vi "Demo_PlotMusic.vi"() -> ()   [LabVIEW 2021, in "RocketPlotDemo.lvlib"]
uses:
  Demo/RocketPlotDemo.lvlib
  TypeDefs/plot load data V2.ctl
  TypeDefs/plot properties V2.ctl
  TypeDefs/plot attributes V2.ctl
  TypeDefs/Plot scale axis properties.ctl
  TypeDefs/Plot general properties.ctl
  Classes/RocketPlotHandle/SubVIs/Init Options.ctl
  TypeDefs/TimeZone.ctl
  Classes/BjusticePlotHandle/Type.ctl
  <vilib>/sound2/lvsound2.llb/Sampling Mode.ctl
  Classes/RocketPlotPanel/RocketPlotPanel.lvclass/RocketPlotPanel.ctl
  4dfea61d-788a-4186-b191-4cde70d6fed2.vi
  966c8643-725a-46bd-9dd0-b91467cf4ddd.vi
  eb0507fd-03f2-4275-8513-22fa9a77d05c.vi
  2cc444ce-eb93-4e53-95b9-bbf802b1ec09.vi
  0323ff41-b8ad-4ed8-8c31-07cadd3001fa.vi
  44d01159-0067-4c41-b020-b8d23d8c44ab.vi
  286f873d-ace6-4cc1-b7d0-d8c3bbebe2d8.vi
  d8c1f50c-a031-4c7b-bbc9-5a9a3e4568ff.vi
  d49b8d8d-7917-4e09-824a-362aaf82a6cf.vi
  35cc1419-e3af-44ec-a6f0-6af3754db062.vi
  Classes/RocketPlotPanel/Read RocketPlotHandle.vi
  <userlib>/bjustice/Ring Buffer for Time Series Data Strict Accessor/Unix time epoch/Unix_Epoch_in_Labview.vi
  0323ff41-b8ad-4ed8-8c31-07cadd3001fa.vi/4c2a6c61-f100-483c-8a49-51e57025a24c.vi
  0323ff41-b8ad-4ed8-8c31-07cadd3001fa.vi/e57bc314-87c7-4952-9bc8-929005dac297.vi
  44d01159-0067-4c41-b020-b8d23d8c44ab.vi/4c2a6c61-f100-483c-8a49-51e57025a24c.vi
  44d01159-0067-4c41-b020-b8d23d8c44ab.vi/e57bc314-87c7-4952-9bc8-929005dac297.vi
  <userlib>/bjustice/Ring Buffer for Time Series Data/API Poly.vi
  <userlib>/bjustice/Ring Buffer for Time Series Data/API/Write Array.vi
  d8c1f50c-a031-4c7b-bbc9-5a9a3e4568ff.vi/f2df9050-0eef-46c6-aff6-3ce3a8893ea5.vi
  35cc1419-e3af-44ec-a6f0-6af3754db062.vi/f2df9050-0eef-46c6-aff6-3ce3a8893ea5.vi
  <userlib>/bjustice/Ring Buffer for Time Series Data/SubVIs/Split Values Array.vi
  <userlib>/bjustice/Ring Buffer for Time Series Data/SubVIs/Replace Values Array Multiple Timestamps.vi
  d8c1f50c-a031-4c7b-bbc9-5a9a3e4568ff.vi/f2df9050-0eef-46c6-aff6-3ce3a8893ea5.vi/63c583a5-c20f-4aba-9c90-661423dee4c4.vi
  d8c1f50c-a031-4c7b-bbc9-5a9a3e4568ff.vi/f2df9050-0eef-46c6-aff6-3ce3a8893ea5.vi/52385341-3d9c-45d2-aff5-e082a4793eb1.vi
  d8c1f50c-a031-4c7b-bbc9-5a9a3e4568ff.vi/f2df9050-0eef-46c6-aff6-3ce3a8893ea5.vi/37f29efa-f142-46b1-a185-f0098a95fbb6.vi
  d8c1f50c-a031-4c7b-bbc9-5a9a3e4568ff.vi/f2df9050-0eef-46c6-aff6-3ce3a8893ea5.vi/84b3d231-9afe-4b6e-afae-e0be43a31e4e.vi
  d8c1f50c-a031-4c7b-bbc9-5a9a3e4568ff.vi/f2df9050-0eef-46c6-aff6-3ce3a8893ea5.vi/c726271c-fc36-4bb7-8553-8945ec40c1cd.vi
  d8c1f50c-a031-4c7b-bbc9-5a9a3e4568ff.vi/f2df9050-0eef-46c6-aff6-3ce3a8893ea5.vi/a7b1d944-dc88-46f5-9d3e-305d46bbe1f6.vi
  d8c1f50c-a031-4c7b-bbc9-5a9a3e4568ff.vi/f2df9050-0eef-46c6-aff6-3ce3a8893ea5.vi/8abc4a6e-a1d2-4e85-879b-517e0ab55733.vi
  d8c1f50c-a031-4c7b-bbc9-5a9a3e4568ff.vi/f2df9050-0eef-46c6-aff6-3ce3a8893ea5.vi/bd347357-b475-4a03-9ac5-3b85ef11aecc.vi
  d8c1f50c-a031-4c7b-bbc9-5a9a3e4568ff.vi/f2df9050-0eef-46c6-aff6-3ce3a8893ea5.vi/391b36e9-a702-45e4-9499-3914f8833a58.vi
  d8c1f50c-a031-4c7b-bbc9-5a9a3e4568ff.vi/f2df9050-0eef-46c6-aff6-3ce3a8893ea5.vi/44155b33-c915-49ce-9e44-a66693aa70dd.vi
  d8c1f50c-a031-4c7b-bbc9-5a9a3e4568ff.vi/f2df9050-0eef-46c6-aff6-3ce3a8893ea5.vi/36977d53-dbe0-4dbc-b2ac-3dea4345b868.vi
  35cc1419-e3af-44ec-a6f0-6af3754db062.vi/f2df9050-0eef-46c6-aff6-3ce3a8893ea5.vi/63c583a5-c20f-4aba-9c90-661423dee4c4.vi
  35cc1419-e3af-44ec-a6f0-6af3754db062.vi/f2df9050-0eef-46c6-aff6-3ce3a8893ea5.vi/52385341-3d9c-45d2-aff5-e082a4793eb1.vi
  35cc1419-e3af-44ec-a6f0-6af3754db062.vi/f2df9050-0eef-46c6-aff6-3ce3a8893ea5.vi/37f29efa-f142-46b1-a185-f0098a95fbb6.vi
  35cc1419-e3af-44ec-a6f0-6af3754db062.vi/f2df9050-0eef-46c6-aff6-3ce3a8893ea5.vi/84b3d231-9afe-4b6e-afae-e0be43a31e4e.vi
  35cc1419-e3af-44ec-a6f0-6af3754db062.vi/f2df9050-0eef-46c6-aff6-3ce3a8893ea5.vi/c726271c-fc36-4bb7-8553-8945ec40c1cd.vi
  35cc1419-e3af-44ec-a6f0-6af3754db062.vi/f2df9050-0eef-46c6-aff6-3ce3a8893ea5.vi/a7b1d944-dc88-46f5-9d3e-305d46bbe1f6.vi
  35cc1419-e3af-44ec-a6f0-6af3754db062.vi/f2df9050-0eef-46c6-aff6-3ce3a8893ea5.vi/8abc4a6e-a1d2-4e85-879b-517e0ab55733.vi
  35cc1419-e3af-44ec-a6f0-6af3754db062.vi/f2df9050-0eef-46c6-aff6-3ce3a8893ea5.vi/bd347357-b475-4a03-9ac5-3b85ef11aecc.vi
  35cc1419-e3af-44ec-a6f0-6af3754db062.vi/f2df9050-0eef-46c6-aff6-3ce3a8893ea5.vi/391b36e9-a702-45e4-9499-3914f8833a58.vi
  35cc1419-e3af-44ec-a6f0-6af3754db062.vi/f2df9050-0eef-46c6-aff6-3ce3a8893ea5.vi/44155b33-c915-49ce-9e44-a66693aa70dd.vi
  35cc1419-e3af-44ec-a6f0-6af3754db062.vi/f2df9050-0eef-46c6-aff6-3ce3a8893ea5.vi/36977d53-dbe0-4dbc-b2ac-3dea4345b868.vi
  <userlib>/bjustice/Ring Buffer for Time Series Data/SubVIs/Enforce array size multiple timestamps.vi
  Classes/BjusticePlotHandle/BjusticePlotHandle.lvclass
  C:/Users/bjustice/Documents/GitHub/BluePlot/Source/Classes/RocketPlotHandle/RocketPlotHandle.lvclass
  Classes/RocketPlotPanel/RocketPlotPanel.lvclass
  C:/Program Files/National Instruments/LabVIEW 2021/vi.lib/IlluminatedG/IG OOPanel/OOPanel/Panel/Panel.lvclass
  <vilib>/sound2/lvsound2.llb/Sound File Info (path).vi
  <vilib>/sound2/lvsound2.llb/Sound File Read Open.vi
  <vilib>/sound2/lvsound2.llb/Sound Output Set Volume (Single).vi
  Classes/RocketPlotHandle/Load PlotConfig.vi
  Classes/RocketPlotHandle/Get PlotConfig.vi
  <vilib>/sound2/lvsound2.llb/Sound File Read (DBL).vi
  <vilib>/Utility/error.llb/Error Cluster From Error Code.vi
  <vilib>/sound2/lvsound2.llb/Sound Output Write (DBL).vi
  Classes/RocketPlotHandle/RocketPlotHandle.lvclass
  RocketPlot.lvlib
  <userlib>/bjustice/Ring Buffer for Time Series Data Strict Accessor/Ring Buffer Strict Accessor.lvlib
  <vilib>/IlluminatedG/IG OOPanel/OOPanel/Manager/Manager.lvclass
panel:
  in  "volume":dbl=100.0
  out "total number of samples/ch":u32
  out "Current Iteration":i32
  out "Current Data":waveform(dbl)[](graph)
  in  "load config":bool
  in  "get config":bool
  out "time to plot":dbl
  out "Subscribed names":i32(listbox)
  in  "Plot config":T1={"plots"=[], "X-axis"={"Name Label.Text"="", "Style"=0, "Tick Colors:Minor Tick Color"=0, "Tick Colors:Tick Color"=0, "Marker Colors:Text Color"=0, "Grid Colors:Major Color"=0, "Grid Colors:Minor Color"=0, "Mapping Mode"=0, "Flipped"=FALSE, "Name Label.Visible"=FALSE, "Name Label.Text Colors:Text Color"=0, "Scale Fit"=0, "Range:Maximum"=0.0, "Range:Minimum"=0.0, "Offset and Multiplier:Multiplier"=0.0, "Offset and Multiplier:Offset"=0.0, "Name Label.Font:Size"=0, "Marker.Font:Size"=0, "Uniform Marker Spacing?"=TRUE, "Format String"=""}, "Y-axes"=[], "General"={"Title"="", "Time to Plot"=1800.0, "Title.Visible"=FALSE, "Sidebar.Visible"=FALSE, "Plot Area:Colors:BG Color"=0, "X Scale.Plot Name"="", "X Scale.Use Plot Name"=FALSE}} {"General"."Time to Plot" format="%<%M:%S>t"}
  # "Documentation and user guide:"
  # "https://github.com/justiceb/BluePlot/blob/main/README.md"
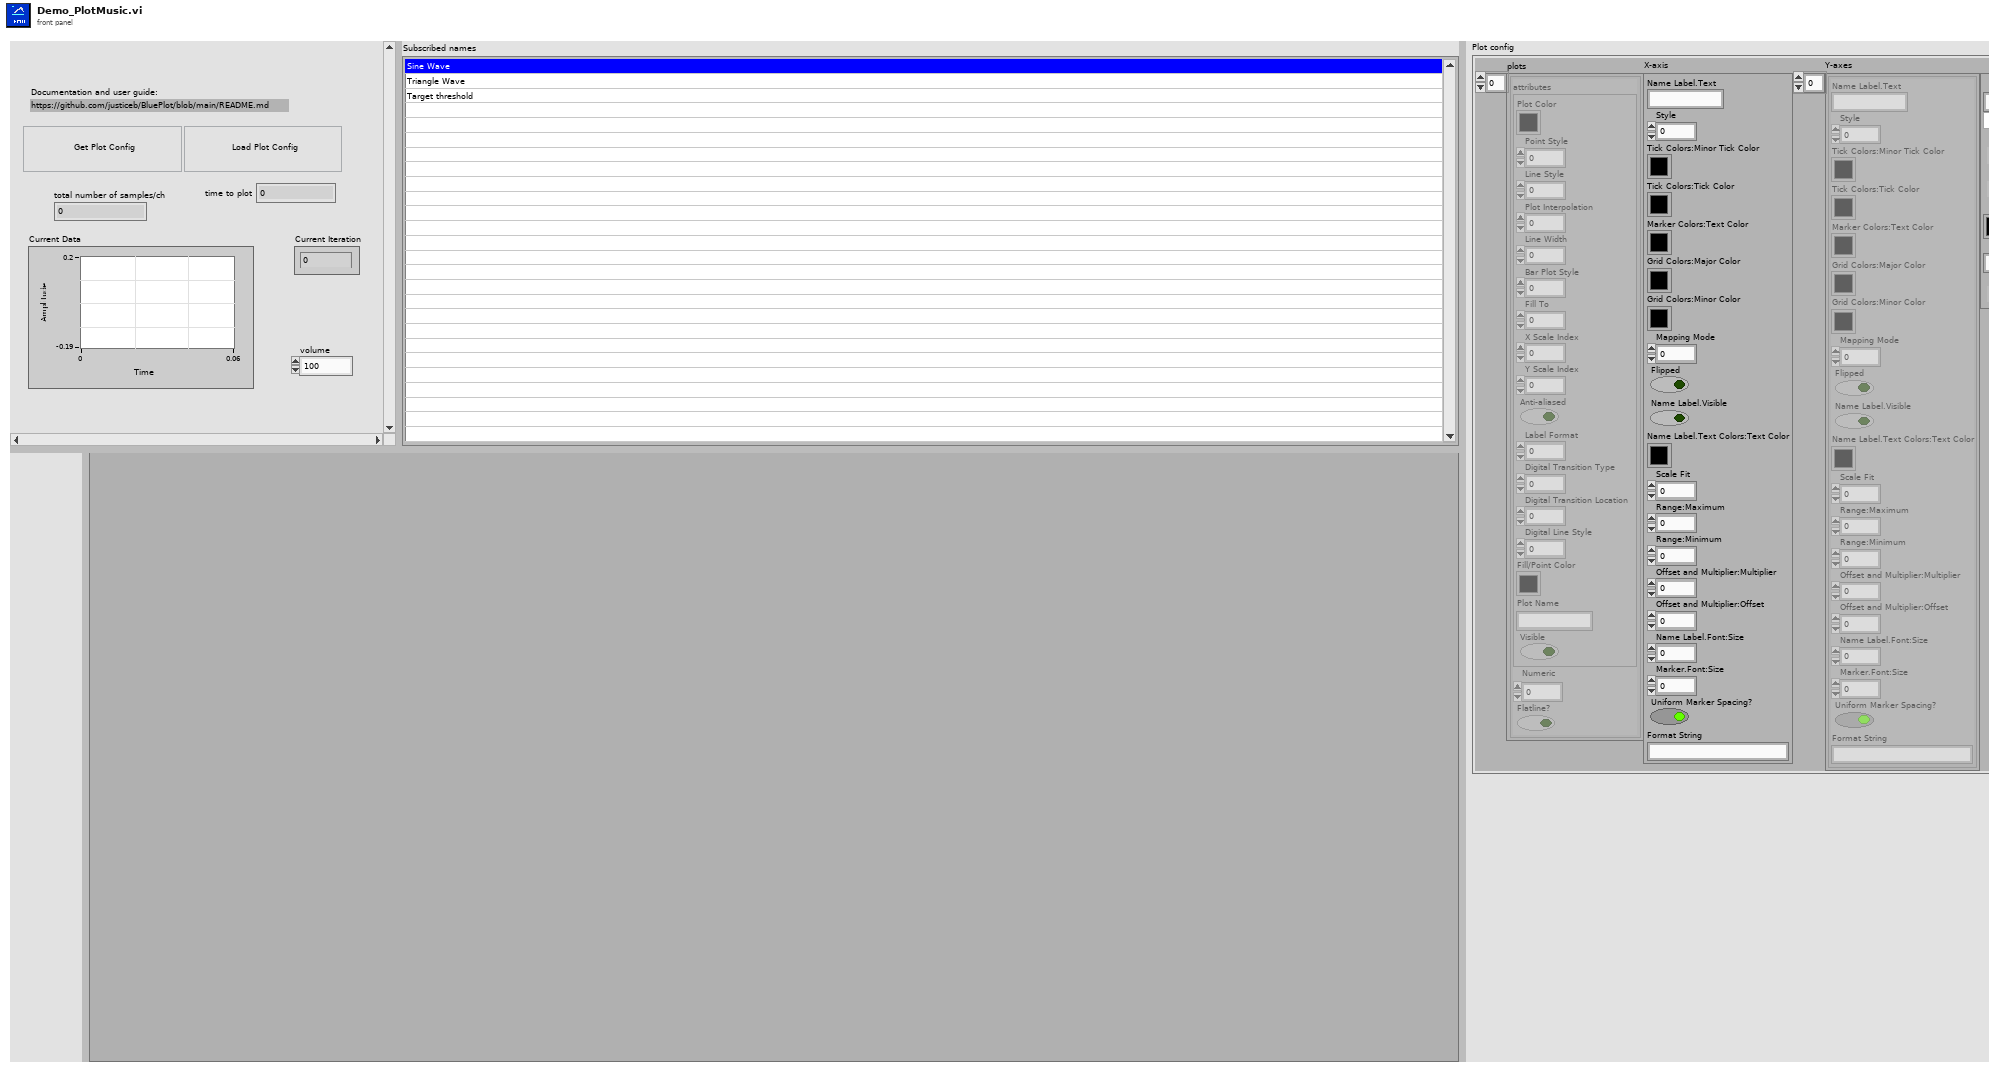
[diagram p1: front panel]
types:
  T1 = typedef "RocketPlot.lvlib/plot load data V2.ctl" = cluster{"plots":T2[], "X-axis":T4, "Y-axes":T4[], "General":T5}
  T2 = typedef "RocketPlot.lvlib/plot properties V2.ctl" = cluster{"attributes":T3, "Numeric":dbl, "Flatline?":bool}
  T3 = typedef "RocketPlot.lvlib/plot attributes V2.ctl" = cluster{"Plot Color":u32, "Point Style":u8, "Line Style":u8, "Plot Interpolation":u8, "Line Width":u8, "Bar Plot Style":u8, "Fill To":i16, "X Scale Index":u32, "Y Scale Index":u32, "Anti-aliased":bool, "Label Format":u8, "Digital Transition Type":u8, "Digital Transition Location":u8, "Digital Line Style":u8, "Fill/Point Color":u32, "Plot Name":string, "Visible":bool}
  T4 = typedef "RocketPlot.lvlib/Plot scale axis properties.ctl" = cluster{"Name Label.Text":string, "Style":u8, "Tick Colors:Minor Tick Color":u32, "Tick Colors:Tick Color":u32, "Marker Colors:Text Color":u32, "Grid Colors:Major Color":u32, "Grid Colors:Minor Color":u32, "Mapping Mode":u8, "Flipped":bool, "Name Label.Visible":bool, "Name Label.Text Colors:Text Color":u32, "Scale Fit":u8, "Range:Maximum":dbl, "Range:Minimum":dbl, "Offset and Multiplier:Multiplier":dbl, "Offset and Multiplier:Offset":dbl, "Name Label.Font:Size":u32, "Marker.Font:Size":u32, "Uniform Marker Spacing?":bool, "Format String":string}
  T5 = typedef "RocketPlot.lvlib/Plot general properties.ctl" = cluster{"Title":string, "Time to Plot":dbl, "Title.Visible":bool, "Sidebar.Visible":bool, "Plot Area:Colors:BG Color":u32, "X Scale.Plot Name":string, "X Scale.Use Plot Name":bool}
  T6 = typedef "Sampling Mode.ctl" = i32
  T7 = typedef "BjusticePlotHandle.lvclass/Type.ctl" = enum16{"1PLOT", "MPLOT"}
  T8 = typedef "RocketPlotHandle.lvclass/Init Options.ctl" = cluster{"UI visible?":bool, "Update rate (ms)":u32, "Sidebar.Visible":bool, "time to plot (init)":dbl, "time to plot (max)":dbl, "config file start path":path, "Title.Visible":bool, "Title":string, "TimeZone":T9}
  T9 = typedef "RocketPlot.lvlib/TimeZone.ctl" = enum16{"UTC", "Local"}
  T10 = typedef "Sound Data Format.ctl" = cluster{"sample rate (S/s)":dbl, "number of channels":i32, "bits per sample":i32}
  T11 = typedef "Ring Buffer Strict Accessor.lvlib/RingBufferHandle.ctl" = cluster{"Ring buffer DVR":refnum<data-value>, "Data Type":T12, "Size(s)":i32[], "Endianess":T13, "Buffer Size (#timestamps) [init]":i32}
  T12 = typedef "Ring Buffer Strict Accessor.lvlib/DataType.ctl" = enum16{"uint8", "uint16", "uint32", "uint64", "int8", "int16", "int32", "int64", "float", "double", "extended"}
  T13 = typedef "Ring Buffer Strict Accessor.lvlib/Endianess.ctl" = enum16{"big-endian", "little-endian"}
  T14 = cluster{"subscribed names":refnum<user-event>, "time to plot":refnum<user-event>}
  T15 = typedef "Sound File Refnum.ctl" = refnum<file>
  T16 = typedef "Sound Output Task ID.ctl" = u32
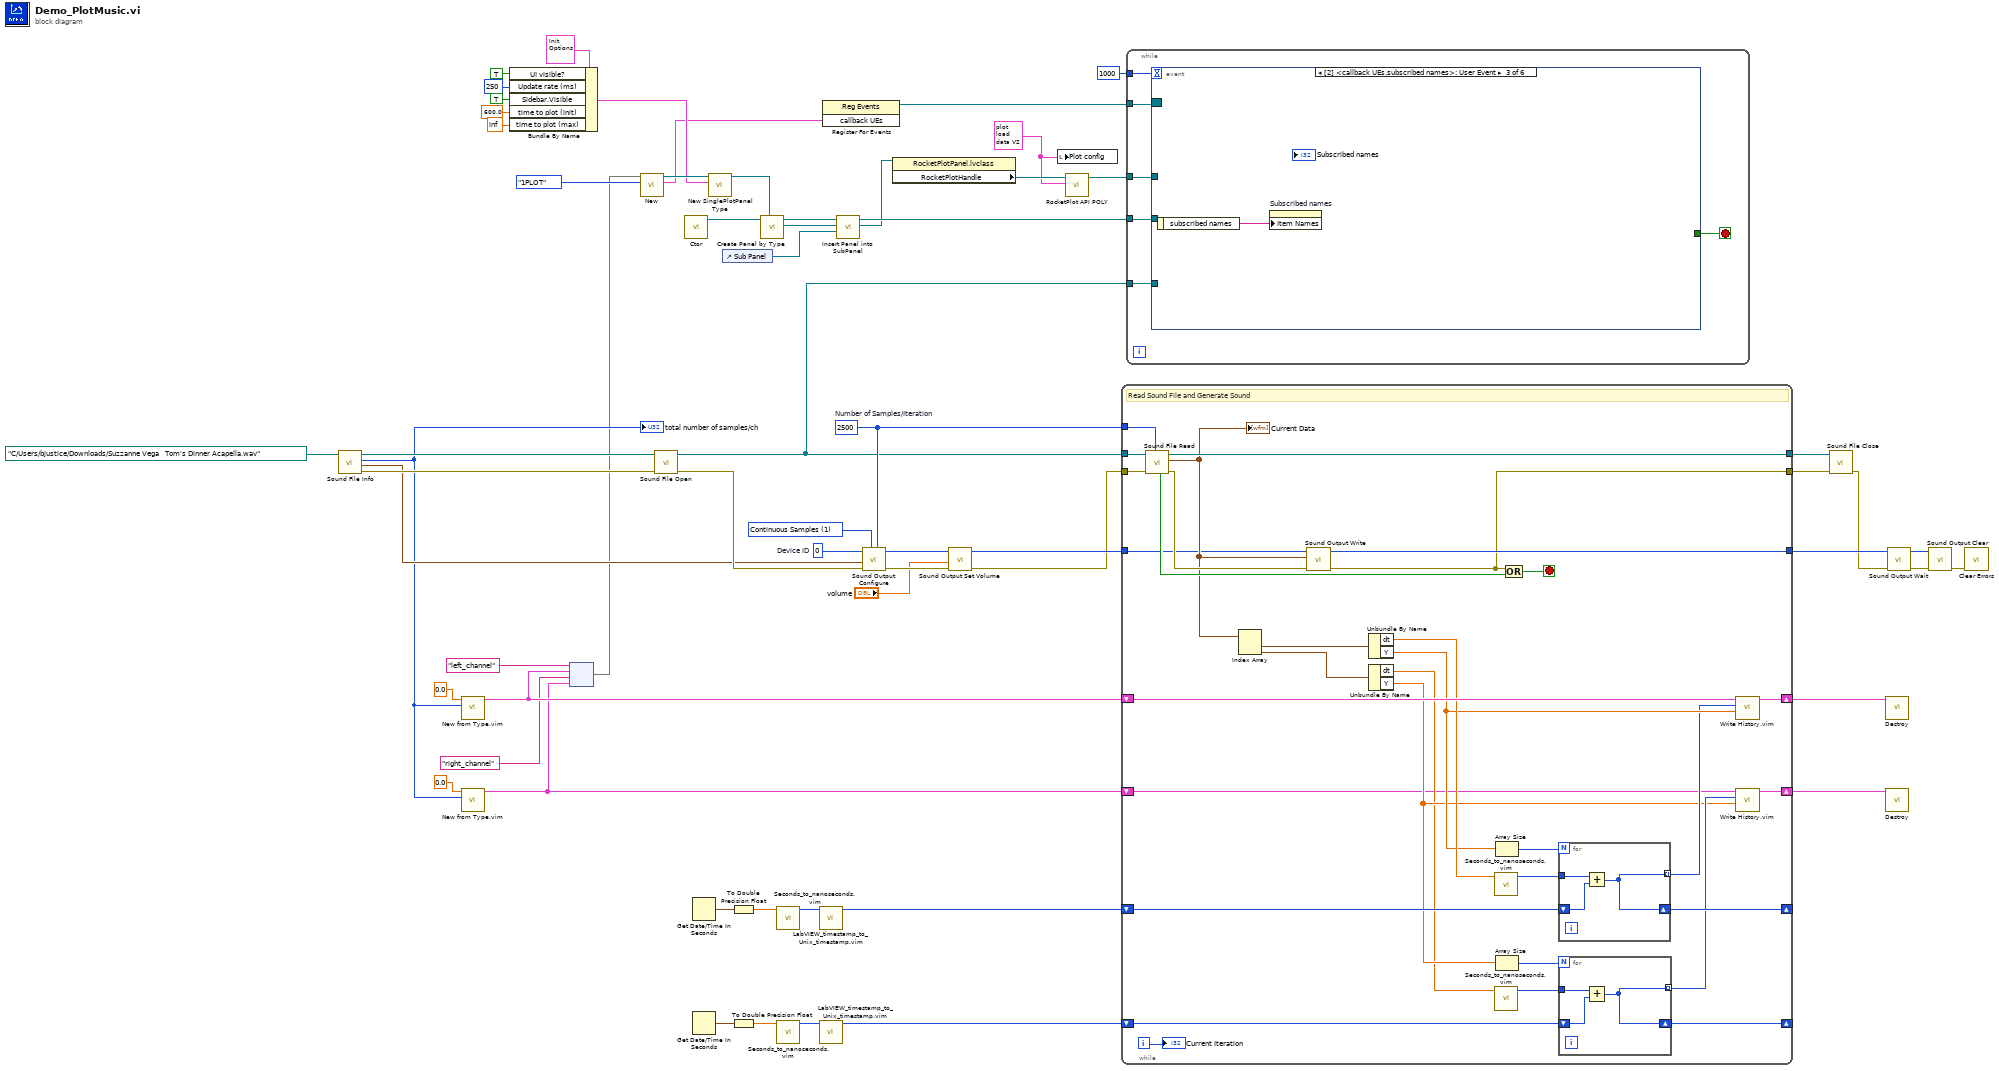
[diagram p0: block diagram]
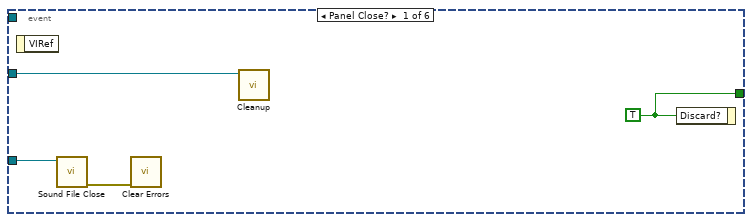
[diagram p2: hidden frame]
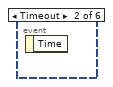
[diagram p3: hidden frame]
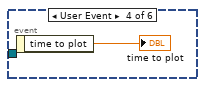
[diagram p4: hidden frame]
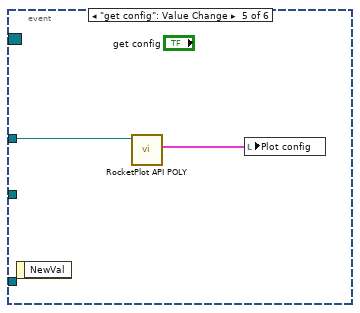
[diagram p5: hidden frame]
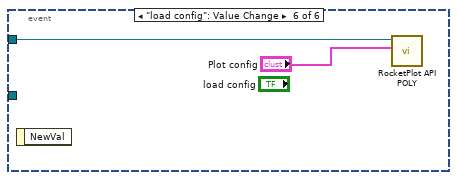
[diagram p6: hidden frame]
diagram:
  w18 = u32 0  # Device ID
  w17 = T6 1 items=["Finite Samples", "Continuous Samples"] ("sample mode")
  w19 = T1 {"plots"=[{"attributes"={"Plot Color"=16711680, "Point Style"=0, "Line Style"=0, "Plot Interpolation"=2, "Line Width"=0, "Bar Plot Style"=0, "Fill To"=-1, "X Scale Index"=0, "Y Scale Index"=0, "Anti-aliased"=FALSE, "Label Format"=3, "Digital Transition Type"=0, "Digital Transition Location"=2, "Digital Line Style"=1, "Fill/Point Color"=16711680, "Plot Name"="left_channel", "Visible"=TRUE}, "Numeric"=0.0, "Flatline?"=FALSE}, {"attributes"={"Plot Color"=4387583, "Point Style"=0, "Line Style"=0, "Plot Interpolation"=2, "Line Width"=0, "Bar Plot Style"=0, "Fill To"=-1, "X Scale Index"=0, "Y Scale Index"=1, "Anti-aliased"=FALSE, "Label Format"=3, "Digital Transition Type"=0, "Digital Transition Location"=2, "Digital Line Style"=1, "Fill/Point Color"=4387583, "Plot Name"="right_channel", "Visible"=TRUE}, "Numeric"=0.0, "Flatline?"=FALSE}, {"attributes"={"Plot Color"=16722671, "Point Style"=0, "Line Style"=0, "Plot Interpolation"=2, "Line Width"=5, "Bar Plot Style"=0, "Fill To"=-1, "X Scale Index"=0, "Y Scale Index"=0, "Anti-aliased"=FALSE, "Label Format"=3, "Digital Transition Type"=0, "Digital Transition Location"=2, "Digital Line Style"=1, "Fill/Point Color"=16722671, "Plot Name"="", "Visible"=TRUE}, "Numeric"=0.0, "Flatline?"=FALSE}], "X-axis"={"Name Label.Text"="Time (s)", "Style"=0, "Tick Colors:Minor Tick Color"=16777216, "Tick Colors:Tick Color"=3684408, "Marker Colors:Text Color"=16448250, "Grid Colors:Major Color"=3684408, "Grid Colors:Minor Color"=16777216, "Mapping Mode"=0, "Flipped"=FALSE, "Name Label.Visible"=TRUE, "Name Label.Text Colors:Text Color"=16448250, "Scale Fit"=2, "Range:Maximum"=3867076442.0, "Range:Minimum"=3867076433.0, "Offset and Multiplier:Multiplier"=1.0, "Offset and Multiplier:Offset"=0.0, "Name Label.Font:Size"=15, "Marker.Font:Size"=15, "Uniform Marker Spacing?"=TRUE, "Format String"="%<%H:%M:%S>T"}, "Y-axes"=[{"Name Label.Text"="Left Axis", "Style"=0, "Tick Colors:Minor Tick Color"=16777216, "Tick Colors:Tick Color"=3684408, "Marker Colors:Text Color"=16448250, "Grid Colors:Major Color"=3684408, "Grid Colors:Minor Color"=16777216, "Mapping Mode"=0, "Flipped"=FALSE, "Name Label.Visible"=FALSE, "Name Label.Text Colors:Text Color"=16448250, "Scale Fit"=2, "Range:Maximum"=0.5, "Range:Minimum"=-0.5, "Offset and Multiplier:Multiplier"=1.0, "Offset and Multiplier:Offset"=0.0, "Name Label.Font:Size"=15, "Marker.Font:Size"=15, "Uniform Marker Spacing?"=TRUE, "Format String"="%#_g"}, {"Name Label.Text"="Right Axis", "Style"=0, "Tick Colors:Minor Tick Color"=16777216, "Tick Colors:Tick Color"=3684408, "Marker Colors:Text Color"=16448250, "Grid Colors:Major Color"=3684408, "Grid Colors:Minor Color"=16777216, "Mapping Mode"=0, "Flipped"=FALSE, "Name Label.Visible"=FALSE, "Name Label.Text Colors:Text Color"=16448250, "Scale Fit"=2, "Range:Maximum"=0.5, "Range:Minimum"=-0.6000000000000001, "Offset and Multiplier:Multiplier"=1.0, "Offset and Multiplier:Offset"=0.0, "Name Label.Font:Size"=15, "Marker.Font:Size"=15, "Uniform Marker Spacing?"=TRUE, "Format String"="%#_g"}], "General"={"Title"="Title", "Time to Plot"=600.0, "Title.Visible"=TRUE, "Sidebar.Visible"=TRUE, "Plot Area:Colors:BG Color"=0, "X Scale.Plot Name"="", "X Scale.Use Plot Name"=FALSE}} ("Plot config 2")
  w54 = 2500  # Number of Samples/Iteration
  n1 = call-poly <vilib>:"Sound File Info.vi"("path"=path "C:/Users/bjustice/Downloads/Suzzanne Vega   Tom's Dinner Acapella.wav") -> ("error out"=w59:errorcluster, "sound format"=w30:T10, "total number of samples/ch"=w20:u32, "path out"=w55:path)  [unwired: 7 in]
  "total number of samples/ch" <- w20
  n2 = call "New from Type.vim"("Buffer Size (#timestamps)"=w20, "LV type (array size cannot be empty)"=0.0 ("value")) -> ("Ring Buffer"=w7:T11)  [unwired: 8 in, 1 out]
  n3 = call "New from Type.vim"("Buffer Size (#timestamps)"=w20, "LV type (array size cannot be empty)"=0.0 ("value")) -> ("Ring Buffer"=w5:T11)  [unwired: 8 in, 1 out]
  n4 = Bundle By Name(cluster=T8 {"UI visible?"=TRUE, "Update rate (ms)"=250, "Sidebar.Visible"=TRUE, "time to plot (init)"=600.0, "time to plot (max)"=inf, "config file start path"=path "", "Title.Visible"=TRUE, "Title"="Title", "TimeZone"=enum."Local"} ("Init options"), "UI visible?"=TRUE, "Update rate (ms)"=u32 250, "Sidebar.Visible"=TRUE ("visible sidebar?"), "time to plot (init)"=600.0, "time to plot (max)"=inf) -> (w41:T8)
  n5 = node("left_channel" ("Name (Read/Add)"), w7, "right_channel" ("Name (Read/Add)"), w5) -> (w1:map{string, T11})
  n6 = call <userlib>:"New.vi"("Type"=Type."1PLOT", "ChannelMap"=w1) -> ("callback UEs"=w2:T14, "StokePlotHandle out"=w42:refnum<class "BjusticePlotHandle.lvclass">)  [unwired: 7 in, 1 out]
  n7 = call-poly <vilib>:"Sound File Open.vi"("error in (no error)"=w59, "path"=w55) -> ("error out"=w58:errorcluster, "sound file refnum"=w21:T15)  [unwired: 8 in]
  n8 = call <vilib>:"Ctor.vi"() -> ("Manager out"=w43:refnum<class "Manager.lvclass">)  [unwired: 10 in, 1 out]
  n9 = Get Date/Time In Seconds() -> (seconds since 1Jan1904=w32:timestamp)
  n10 = Get Date/Time In Seconds() -> (seconds since 1Jan1904=w25:timestamp)
  n11 = call "New SinglePlotPanel Type.vi"("Init options"=w41, "BluePlotHandle"=w42) -> ("SinglePlotPanel out"=w40:refnum<class "RocketPlotPanel.lvclass">)  [unwired: 8 in, 1 out]
  n12 = control-ref of="Sub Panel"() -> (w38:refnum<vi>)
  n13 = To Double Precision Float(number=w32) -> (double precision float=w31:dbl)
  n14 = To Double Precision Float(number=w25) -> (double precision float=w26:dbl)
  n15 = call <vilib>:"Create Panel by Type.vi"("Panel Type"=w40, "Manager in"=w43) -> ("Panel"=w37:refnum<class "RocketPlotPanel.lvclass">, "Manager out"=w39:refnum<class "Manager.lvclass">)  [unwired: 7 in, 1 out]
  n16 = call "Seconds_to_nanoseconds.vim"("timestamp (seconds)"=w31) -> ("timestamp (nanoseconds)"=w34:u64)  [unwired: 10 in]
  n17 = call "Seconds_to_nanoseconds.vim"("timestamp (seconds)"=w26) -> ("timestamp (nanoseconds)"=w24:u64)  [unwired: 10 in]
  n18 = call "LabVIEW_timestamp_to_Unix_timestamp.vim"("LabVIEW timestamp (nanoseconds)"=w34) -> ("Unix timestamp (nanoseconds)"=w28:u64)  [unwired: 10 in]
  n19 = call "LabVIEW_timestamp_to_Unix_timestamp.vim"("LabVIEW timestamp (nanoseconds)"=w24) -> ("Unix timestamp (nanoseconds)"=w27:u64)  [unwired: 10 in]
  n20 = register-events(w2) -> (reference out=w52:refnum<event-registration>)  [unwired: 2 in, 1 out]
  n21 = call <vilib>:"Insert Panel into SubPanel.vi"("SubPanel"=w38, "Panel In"=w37, "Manager in"=w39) -> ("Panel"=w3:refnum<class "RocketPlotPanel.lvclass">, "Manager out"=w35:refnum<class "Manager.lvclass">)  [unwired: 6 in, 1 out]
  n22 = call <vilib>:"Sound Output Configure.vi"("number of samples/ch"=w54, "sample mode"=w17, "error in (no error)"=w58, "sound format"=w30, "device ID"=w18) -> ("error out"=w12:errorcluster, "task ID"=w13:T16)  [unwired: 5 in]
  n23 = property class="RocketPlotPanel.lvclass"(reference=w3) -> ("RocketPlotHandle"=w36:refnum<class "RocketPlotHandle.lvclass">)  [unwired: 1 in, 2 out]
  n24 = call-poly <vilib>:"Sound Output Set Volume.vi"("error in (no error)"=w12, "volume"="volume", "task ID"=w13) -> ("error out"=w10:errorcluster, "task ID out"=w11:T16)  [unwired: 7 in]
  n25 = local write "Plot config"(w19) -> ()
  n26 = call-poly "RocketPlot API POLY.vi"("Plot config"=w19, "BluePlotHandle in"=w36) -> ("BluePlotHandle out"=w45:refnum<class "RocketPlotHandle.lvclass">)  [unwired: 8 in, 1 out]
  n27 = while {
    tunnel: w54 -> [w85]
    tunnel: w21 -> [w91]
    tunnel: [w89] -> w61
    tunnel: w10 -> [w92]
    tunnel: [w84] -> w60
    tunnel: [w93] -> w57
    shift-right: [w74] -> _
    shift-left: w28 -> [w76]
    shift-right: [w73] -> _
    shift-left: w27 -> [w71]
    shift-right: [w64] -> w23
    shift-left: w7 -> [w82]
    shift-right: [w63] -> w22
    shift-left: w5 -> [w66]
    tunnel: w11 -> [w62]
    i -> [w90]
    stop <- w86 stop-if-true
    # "Read Sound File and Generate Sound"
    n28 = call-poly <vilib>:"Sound File Read.vi"("number of samples/ch (-1: all)"=w85, "error in (no error)"=w92, "sound file refnum"=w91) -> ("error out"=w88:errorcluster, "data"=w83:waveform(dbl)[], "sound file refnum out"=w89:T15, "end of file?"=w87:bool)  [unwired: 4 in, 1 out]
    "Current Data" <- w83
    n29 = Index Array(array=w83) -> (element #1=w81:waveform(dbl), element #2=w65:waveform(dbl))  [unwired: 2 in]
    n30 = call-poly <vilib>:"Sound Output Write.vi"("error in (no error)"=w88, "data"=w83, "task ID"=w62) -> ("error out"=w84:errorcluster, "task ID out"=w93:T16)  [unwired: 7 in]
    n31 = Unbundle By Name(w81) -> ("dt"=w80:dbl, "Y"=w79:dbl[])
    n32 = Unbundle By Name(w65) -> ("dt"=w67:dbl, "Y"=w68:dbl[])
    n33 = call "Seconds_to_nanoseconds.vim"("timestamp (seconds)"=w80) -> ("timestamp (nanoseconds)"=w77:u64)  [unwired: 10 in]
    n34 = call "Seconds_to_nanoseconds.vim"("timestamp (seconds)"=w67) -> ("timestamp (nanoseconds)"=w70:u64)  [unwired: 10 in]
    n35 = Array Size(array=w79) -> (size(s)=w78:i32)
    n36 = Array Size(array=w68) -> (size(s)=w69:i32)
    n37 = Compound Arithmetic op=OR(w84, w87) -> (w86:bool)
    n38 = for {
      N: w78 -> [_]
      tunnel: w77 -> [w96]
      shift-right: [w94] -> w74
      shift-left: w76 -> [w95]
      tunnel: [w94] -> w75 mode=indexing
      n39 = Add(x=w96, y=w95) -> (x+y=w94:u64)
    }
    n40 = for {
      N: w69 -> [_]
      tunnel: w70 -> [w99]
      shift-right: [w97] -> w73
      shift-left: w71 -> [w98]
      tunnel: [w97] -> w72 mode=indexing
      n41 = Add(x=w99, y=w98) -> (x+y=w97:u64)
    }
    n42 = call "Write History.vim"("LV DataType"=w79, "Timestamps"=w75, "Ring Buffer"=w82) -> ("Ring Buffer"=w64:T11)  [unwired: 7 in, 1 out]
    n43 = call "Write History.vim"("LV DataType"=w68, "Timestamps"=w72, "Ring Buffer"=w66) -> ("Ring Buffer"=w63:T11)  [unwired: 7 in, 1 out]
    "Current Iteration" <- w90
  }
  n44 = while {
    tunnel: w45 -> [w105]
    tunnel: w52 -> [w103]
    tunnel: 1000 ("period (ms)") -> [w102]
    tunnel: w35 -> [w101]
    tunnel: w21 -> [w100]
    stop <- w104 stop-if-true
    n45 = event shown="[2] <callback UEs.subscribed names>: User Event" {
      selector: w103 -> [_ _ _ _ _ _]
      dyn-events: _ -> [_ _ _ _ _ _]
      timeout: w102 -> [_ _ _ _ _ _]
      tunnel: w105 -> [_ _ _ _ w113 w115]
      tunnel: [w109 _ _ _ _ _] -> w104
      tunnel: w101 -> [w108 _ _ _ _ _]
      tunnel: w100 -> [w107 _ _ _ _ _]
      event Panel Close? {
        w109 = TRUE ("Discard?")
        n46 = event-data() -> ()  [unwired: 1 in, 1 out]
        n47 = call <vilib>:"Sound File Close.vi"("sound file refnum"=w107) -> ("error out"=w106:errorcluster)  [unwired: 10 in]
        n48 = call <vilib>:"Clear Errors.vi"("error in (no error)"=w106) -> ()  [unwired: 5 in, 2 out]
        n49 = call <vilib>:"Cleanup.vi"("Manager in"=w108) -> ()  [unwired: 8 in, 3 out]
        n50 = event-data("Discard?"=w109) -> ()  [unwired: 1 in, 1 out]
      }
      event Timeout {
        n51 = event-data() -> ()  [unwired: 1 in, 1 out]
      }
      event User Event {
        n52 = event-data() -> ("subscribed names"=w110:string[])  [unwired: 1 in]
        n53 = property on="Subscribed names" class="LstBox (strict)"("Item Names"=w110) -> ()  [unwired: 2 in, 2 out]
      }
      event User Event {
        n54 = event-data() -> ("time to plot"=→"time to plot":dbl)  [unwired: 1 in]
      }
      event "get config": Value Change {
        n55 = event-data() -> ()  [unwired: 1 in, 1 out]
        n56 = call-poly "RocketPlot API POLY.vi"("BluePlotHandle in"=w113) -> ("Plot config"=w112:T1)  [unwired: 8 in, 2 out]
        n57 = local write "Plot config"(w112) -> ()
      }
      event "load config": Value Change {
        n58 = event-data() -> ()  [unwired: 1 in, 1 out]
        n59 = call-poly "RocketPlot API POLY.vi"("Plot config"="Plot config", "BluePlotHandle in"=w115) -> ()  [unwired: 8 in, 2 out]
      }
    }
  }
  n60 = call <vilib>:"Sound File Close.vi"("error in (no error)"=w60, "sound file refnum"=w61) -> ("error out"=w56:errorcluster)  [unwired: 9 in]
  n61 = call <userlib>:"Destroy.vi"("Ring Buffer"=w23) -> ()  [unwired: 10 in, 1 out]
  n62 = call <userlib>:"Destroy.vi"("Ring Buffer"=w22) -> ()  [unwired: 10 in, 1 out]
  n63 = call <vilib>:"Sound Output Wait.vi"("error in (no error)"=w56, "task ID"=w57) -> ("error out"=w15:errorcluster, "task ID out"=w16:T16)  [unwired: 8 in]
  n64 = call <vilib>:"Sound Output Clear.vi"("error in (no error)"=w15, "task ID"=w16) -> ("error out"=w14:errorcluster)  [unwired: 9 in]
  n65 = call <vilib>:"Clear Errors.vi"("error in (no error)"=w14) -> ()  [unwired: 5 in, 2 out]
